vi "Actor Core.vi"(8 "error in":errorcluster, 11 "Lock-in in":refnum<class "Lock-in.lvclass">) -> (0 "error out":errorcluster, 3 "Actor out":refnum<class "Actor.lvclass">)   [LabVIEW 2018, in "Lock-in.lvclass"]
doc: "(<B>Filename</B>: Actor Framework.lvlib:Actor.lvclass:Actor Core.vi)\n\nReceives messages to the actor, reacts to them, and initiates any error handling that may shut the actor down.\n\nDescendant classes may override this VI to append parallel tasks for the actor to complete while it handles messages. Overrides use the Call Parent Method node."
uses:
  Lock-in.lvclass
  C:/github/LabActor/Template Module/Template Module.lvclass
  C:/Program Files/National Instruments/LabVIEW 2018/vi.lib/ActorFramework/Actor/Actor.lvclass
  <vilib>/ActorFramework/Actor/Actor.lvclass
  NHMFL_Core/Libraries/Instruments/Instrument Driver/Lock-in Driver/Lock-in Configuration.ctl
  Lock-in.lvclass/Lock-in.ctl
  Template Module/Template Module.lvclass/Template Module.ctl
  <vilib>/ActorFramework/Actor/Actor.lvclass/Actor.ctl
  <vilib>/ActorFramework/Message Enqueuer/Message Enqueuer.lvclass/Message Enqueuer.ctl
  Lock-in Messages/Set Frequency Msg/Set Frequency Msg.lvclass/Set Frequency Msg.ctl
  Template Module/Read stop event.vi
  <vilib>/ActorFramework/Message Enqueuer/Init from Existing Queue.vi
  <vilib>/ActorFramework/Message Enqueuer/Enqueue.vi
  Lock-in Messages/Set Frequency Msg/Set Frequency Msg.lvclass
  C:/Program Files/National Instruments/LabVIEW 2018/vi.lib/ActorFramework/Message/Message.lvclass
  <vilib>/ActorFramework/Message Priority Queue/Priority Enqueue.vi
  Instrument Actor/Instrument Actor.lvclass
  <vilib>/ActorFramework/Message Enqueuer/Message Enqueuer.lvclass
panel:
  out "Name":string
  in  "Configuration":T1={"Frequency"=100000.0, "Time constant"=1.0, "Synchronous"=FALSE, "Channels"=[1]} {"Time constant" format="%#_6ps"; "Frequency" format="%#_6pHz"}
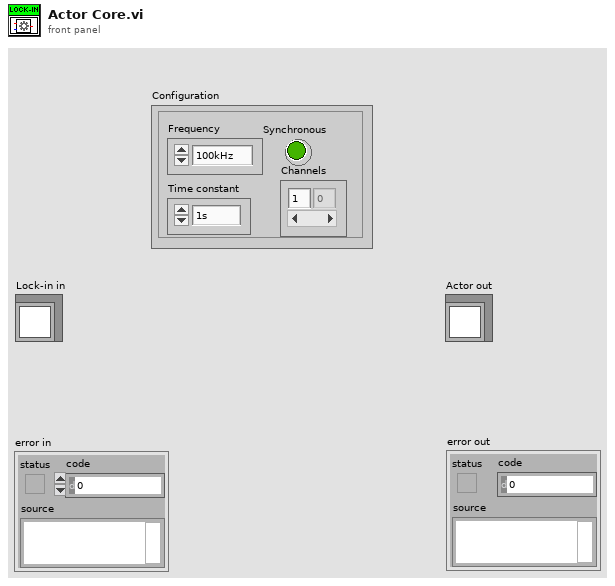
[diagram p1: front panel]
types:
  T1 = typedef "Lock-in Configuration.ctl" = cluster{"Frequency":dbl, "Time constant":dbl, "Synchronous":bool, "Channels":i32[]}
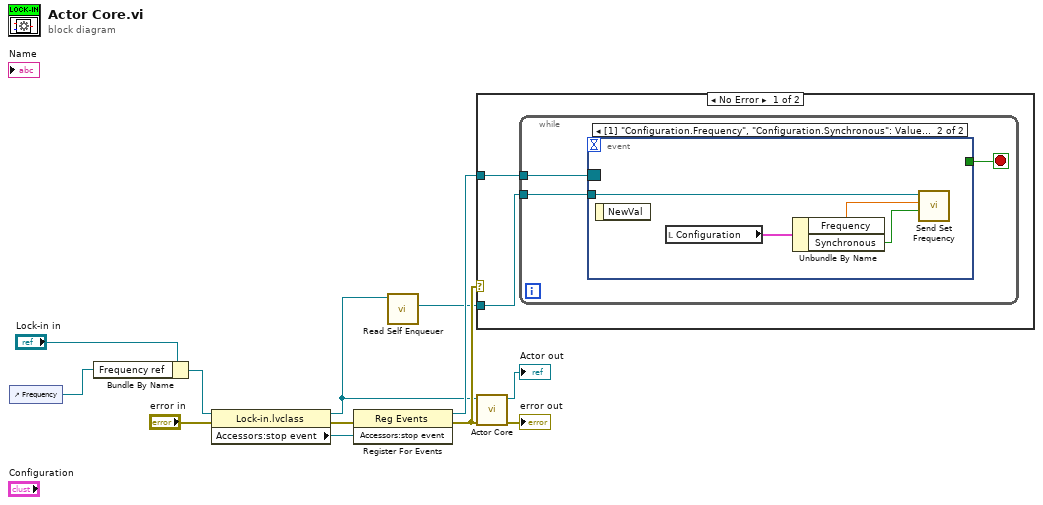
[diagram p0: block diagram]
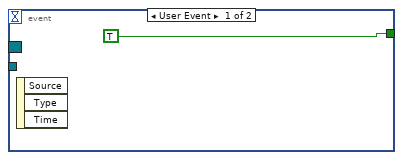
[diagram p2: hidden frame]
diagram:
  n1 = control-ref of="Frequency"() -> (w1:refnum<vi>)
  n2 = Bundle By Name(cluster="Lock-in in", "Frequency ref"=w1) -> (w2:refnum<class "Lock-in.lvclass">)
  n3 = property class="Lock-in.lvclass"(reference=w2, error in="error in") -> (reference out=w4:refnum<class "Lock-in.lvclass">, error out=w6:errorcluster, "Accessors:stop event"=w9:refnum<user-event>)
  n4 = register-events(error in=w6, w9) -> (reference out=w8:refnum<event-registration>, error out=w5:errorcluster)  [unwired: 1 in]
  n5 = call <vilib>:"Read Self Enqueuer.vi"("Actor"=w4) -> ("Self Enqueuer"=w3:refnum<class "Message Enqueuer.lvclass">)  [unwired: 10 in]
  n6 = case shown="No Error" w5 {
    tunnel: w8 -> [w14 _]
    tunnel: w3 -> [w13 _]
    frame No Error {
      n7 = while {
        tunnel: w14 -> [w17]
        tunnel: w13 -> [w15]
        stop <- w16 stop-if-true
        n8 = event shown="[1] \"Configuration.Frequency\", \"Configuration.Synchronous\": Value Change" {
          selector: w17 -> [_ _]
          dyn-events: _ -> [_ _]
          timeout: _ -> [_ _]
          tunnel: [TRUE _] -> w16
          tunnel: w15 -> [_ w22]
          event User Event {
            n9 = event-data() -> ()  [unwired: 1 in, 3 out]
          }
          event Value Change {
            n10 = event-data() -> ()  [unwired: 1 in, 1 out]
            n11 = local read "Configuration"() -> (w21:T1)
            n12 = Unbundle By Name(w21) -> ("Frequency"=w19:dbl, "Synchronous"=w20:bool)
            n13 = call "Send Set Frequency.vi"("Synchronous"=w20, "Frequency"=w19, "Message Enqueuer"=w22) -> ()  [unwired: 7 in, 2 out]
          }
        }
      }
    }
    frame Error {
    }
  }
  n14 = call-parent "Actor Core.vi"("error in"=w5, "Measure Object in"=w4) -> ("error out"=→"error out":errorcluster, "Actor out"=→"Actor out":refnum<class "Actor.lvclass">)  [unwired: 8 in]
